vi "Campionamento Plot.vi"(5 "file path out (dialog if empty)":path, 6 "External File?":bool, 7 "file path (dialog if empty)":path, 10 "Num Max":dbl=100.0, 11 "Spectrum In":dbl[][](array[numeric])) -> (3 "Spectrum Out":dbl[][](array[numeric]))   [LabVIEW 2023]
uses:
  <vilib>/Utility/file.llb/Read Delimited Spreadsheet (DBL).vi
  <vilib>/Utility/file.llb/Write Delimited Spreadsheet (DBL).vi
panel:
  out "XY Graph":cluster{dbl[], dbl[]}[](graph)
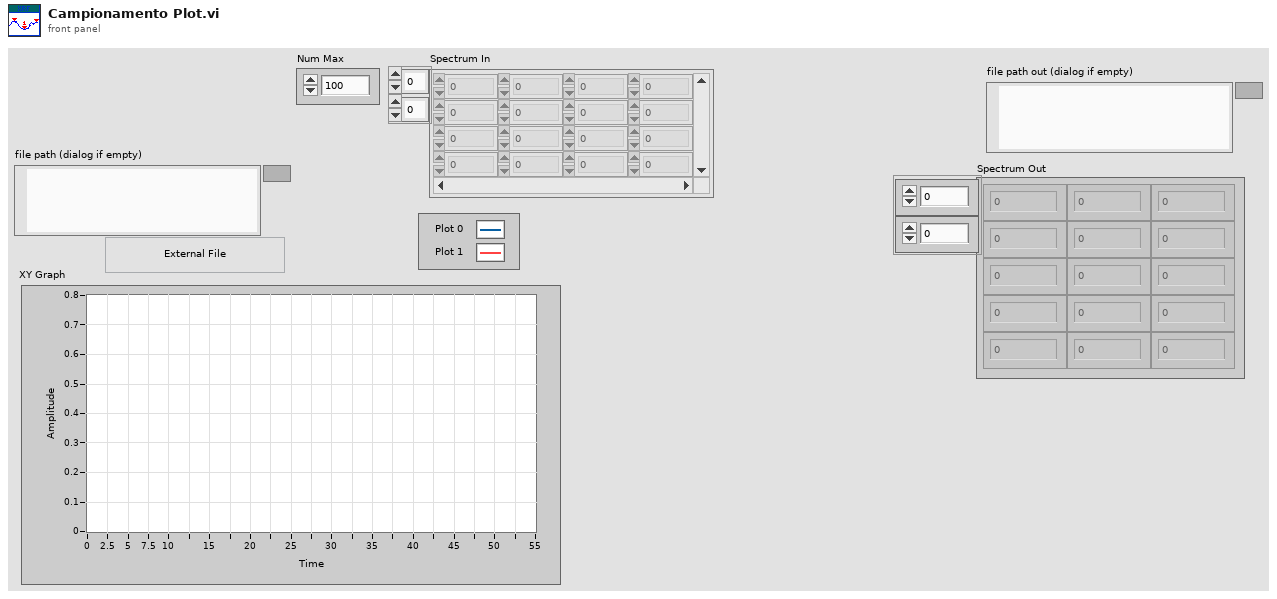
[diagram p1: front panel]
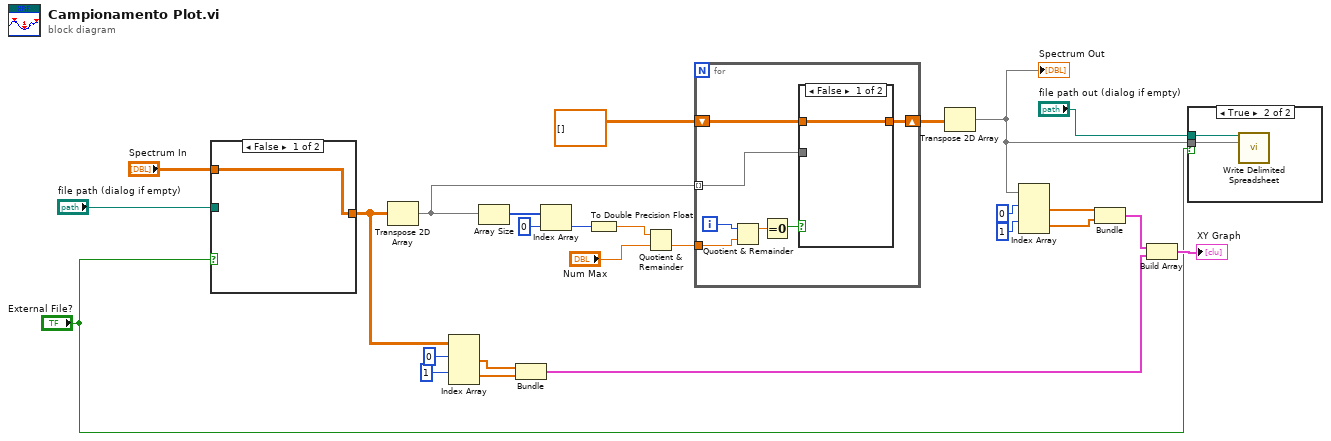
[diagram p0: block diagram]
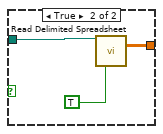
[diagram p3: hidden frame]
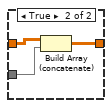
[diagram p4: hidden frame]
diagram:
  n1 = case shown="False" "External File?" {
    tunnel: [w27 w29] -> w4
    tunnel: "file path (dialog if empty)" -> [_ w28]
    tunnel: "Spectrum In" -> [w27 _]
    frame False {
    }
    frame True {
      n2 = call-poly <vilib>:"Read Delimited Spreadsheet.vi"("file path (dialog if empty)"=w28, "transpose? (F)"=TRUE) -> ("all rows"=w29:dbl[][])  [unwired: 8 in, 5 out]
    }
  }
  n3 = Transpose 2D Array(2D array=w4) -> (transposed array=w3:dbl[][])
  n4 = Index Array(array=w4, index (row) #1=0 ("disabled index (col)"), index (row) #2=1 ("index (col)")) -> (element #1=w19:dbl[], element #2=w18:dbl[])  [unwired: 2 in]
  n5 = Array Size(array=w3) -> (size(s)=w26:i32[])
  n6 = Bundle("all rows"=w19, "all rows"=w18) -> (w13:cluster{"all rows":dbl[], "all rows":dbl[]})  [unwired: 1 in]
  n7 = Index Array(array=w26, index=0) -> (element=w24:i32)
  n8 = To Double Precision Float(number=w24) -> (double precision float=w23:dbl)
  n9 = Quotient & Remainder(x=w23, y="Num Max") -> (floor(x/y)=w20:dbl)  [unwired: 1 out]
  n10 = for {
    tunnel: w3 -> [w31] mode=indexing
    shift-right: [w33] -> w2
    shift-left: dbl[][] [] -> [w32]
    tunnel: w20 -> [w36]
    i -> [w37]
    n11 = Quotient & Remainder(x=w37, y=w36) -> (x-y*floor(x/y)=w35:dbl)  [unwired: 1 out]
    n12 = Equal To 0?(x=w35) -> (x = 0?=w34:bool)
    n13 = case shown="False" w34 {
      tunnel: [w38 w39] -> w33
      tunnel: w32 -> [w38 w41]
      tunnel: w31 -> [_ w40]
      frame False {
      }
      frame True {
        n14 = Build Array (concatenate)(w41, w40) -> (w39:dbl[][])
      }
    }
  }
  n15 = Transpose 2D Array(2D array=w2) -> (transposed array=w1:dbl[][])
  "Spectrum Out" <- w1
  n16 = Index Array(array=w1, index (row) #1=0 ("disabled index (col)"), index (row) #2=1 ("index (col)")) -> (element #1=w17:dbl[], element #2=w16:dbl[])  [unwired: 2 in]
  n17 = Bundle(w17, w16) -> (w14:cluster{dbl[], dbl[]})  [unwired: 1 in]
  n18 = Build Array(w14, w13) -> (→"XY Graph":cluster{"all rows":dbl[], "all rows":dbl[]}[])
  n19 = case shown="True" "External File?" {
    tunnel: w1 -> [_ w43]
    tunnel: "file path out (dialog if empty)" -> [_ w42]
    frame False {
    }
    frame True {
      n20 = call-poly <vilib>:"Write Delimited Spreadsheet.vi"("file path (dialog if empty)"=w42, "2D data"=w43) -> ()  [unwired: 12 in, 2 out]
    }
  }
